vi "SamplingRate.vi"() -> ()   [LabVIEW 2013]
panel:
  in  "SamplingRate":i32=5000
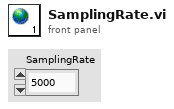
[diagram p1: front panel]
diagram:
